vi "Voltech PM1000+ Inrush Measurement.vi"() -> ()   [LabVIEW 2015]
doc: "The purpose of this vi is to show the basic measurements that PM1000+ can make. The results are returned using the FRD command. This returns the results that are shown on the screen, in the order in which they appear on the screen. As results are selected using comms, the results are added to the bottom of the list, with the exception of harmonics, which always appear at the end of the list."
uses:
  <vilib>/Utility/error.llb/DialogType.ctl
  <instrlib>/Voltech PM1000+/Voltech PM1000+.lvlib
panel:
  in  "Reset (True)":bool=TRUE
  in  "ID Query (True)":bool=TRUE
  in  "Serial Configuration":T1={"Baud Rate"=19200, "Parity"=0, "Data Bits"=8, "Stop Bits"=10, "Flow Control"=2} {"Flow Control" items=["None"=0, "RTS/CTS"=2]; "Stop Bits" items=["1.0"=10]; "Data Bits" items=["8"=8]; "Parity" items=["None"]; "Baud Rate" items=["9600"=9600, "19200"=19200, "38400"=38400]}
  in  "Measurements":T2={"Current Range (100Apk)"=3, "Measurements - Inrush"=[2, 3, 4, 5]} {"Current Range (100Apk)" items=["0.1Apk", "0.4Apk", "1.6Apk", "6.25Apk", "25Apk", "100Apk"]}
  out "Number of Measurements":u32
  in  "Select Mode (Normal)":u16(ring)=2 items=["Normal", "Ballast", "Inrush", "Standby Power", "Integrator"]
  in  "Enable Autozero  (True)":bool=TRUE caption="Autozero  (Enable)"
  in  "Enable Blanking (True)":bool=TRUE
  in  "Shunt (Internal)":u16(ring) items=["Internal", "External"]
  in  "Freq Source (Voltage)":u16(ring) items=["Voltage", "Current"]
  in  "Fixed/Auto Ranging":T3 {"Volts Ranging (Auto)" items=["Auto", "10Vpk", "46Vpk", "215Vpk", "900Vpk"]; "Amps Ranging (Auto)" items=["Auto", "0.1Apk", "0.4Apk", "1.6Apk", "6.25Apk", "25Apk", "100Apk"]}
  in  "Scaling":T4={"Voltage Sacling (1.0000)"=1.0, "Current Sacling (1.0000)"=1.0} {"Current Sacling (1.0000)" min=1e-06 max=1000000.0 step=1.0 format="%.6f"; "Voltage Sacling (1.0000)" min=1e-06 max=1000000.0 step=1.0 format="%.6f"}
  in  "VISA resource name":refnum<visa-resource-name>
  in  "stop":bool
  out "Parameter":string[](array[string])
  out "Value":dbl[](array[numeric])
  # "(c) 2008-2009 Voltech Instruments.  ALL RIGHTS RESERVED."
  # "Configuration Side"
  # "1. Leave it as default or set up the PM1000+ instruments on the left  \n    \"Configuration Side\".\n2. Press Ctrl+R to run the test.\n3. Press the lower right side \"STOP\" button to stop the test."
  # "Results Side"
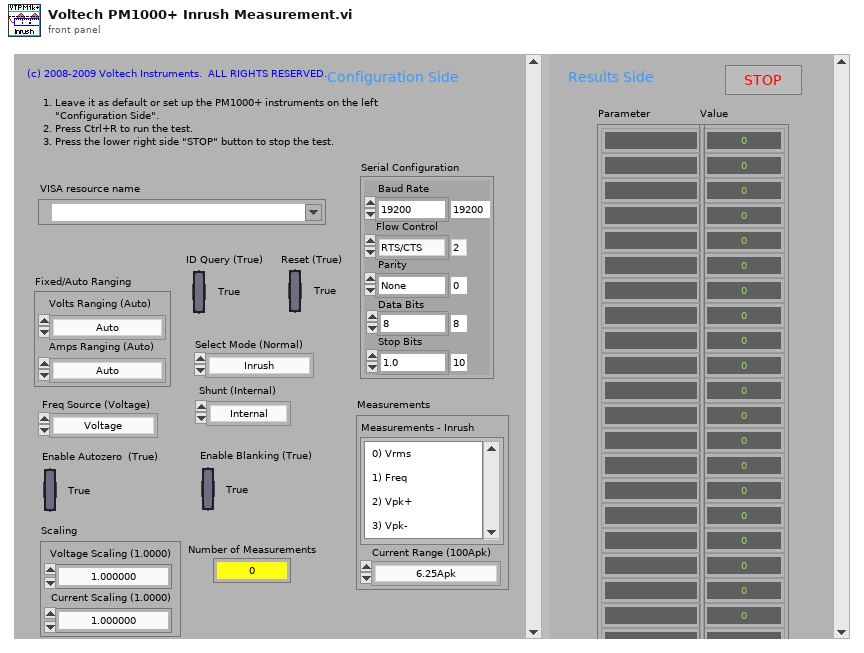
[diagram p1: front panel]
types:
  T1 = cluster{"Baud Rate":u32, "Parity":u16, "Data Bits":u16, "Stop Bits":u16, "Flow Control":u16}
  T2 = cluster{"Current Range (100Apk)":i32, "Measurements - Inrush":i32[]}
  T3 = cluster{"Amps Ranging (Auto)":u16, "Volts Ranging (Auto)":u16}
  T4 = cluster{"Voltage Sacling (1.0000)":dbl, "Current Sacling (1.0000)":dbl}
  T5 = typedef "DialogType.ctl" = u16
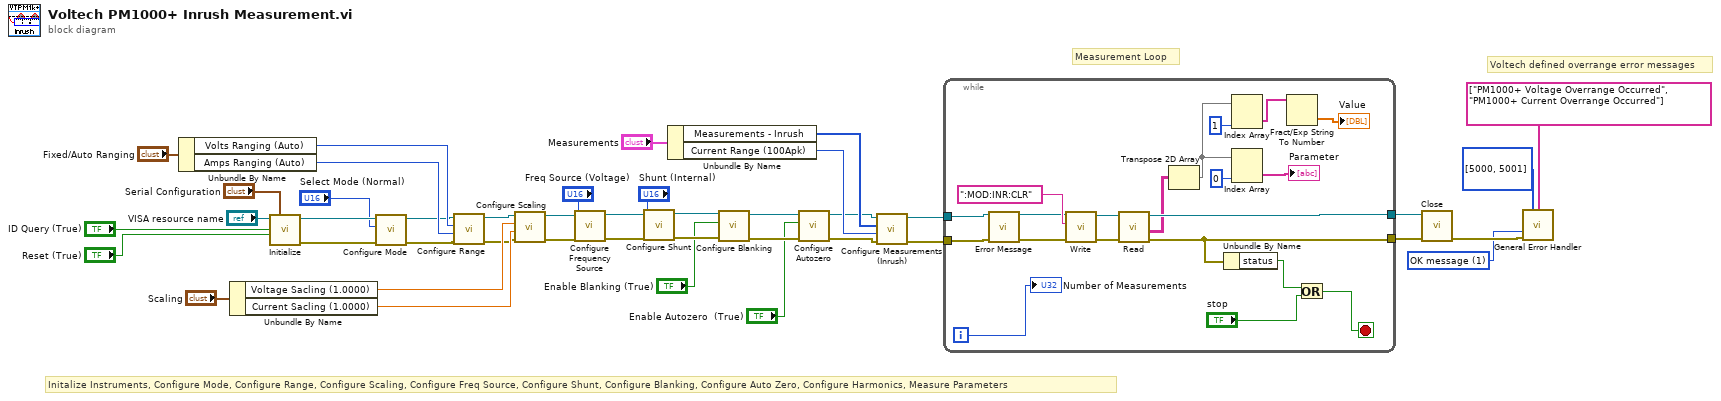
[diagram p0: block diagram]
diagram:
  w14 = T5 1 items=["no dialog", "OK message", "continue or stop message", "OK message + warnings", "continue/stop + warnings"] ("type of dialog (OK msg:1)")
  # "Voltech defined overrange error messages"
  # "Measurement Loop"
  # "Initalize Instruments, Configure Mode, Configure Range, Configure Scaling, Configure Freq Source, Configure Shunt, Configure Blanking, Configure Auto Zero, Configure Harmonics, Measure Parameters"
  n1 = Unbundle By Name("Fixed/Auto Ranging") -> ("Volts Ranging (Auto)"=w29:u16, "Amps Ranging (Auto)"=w28:u16)
  n2 = Unbundle By Name("Scaling") -> ("Voltage Sacling (1.0000)"=w32:dbl, "Current Sacling (1.0000)"=w31:dbl)
  n3 = call <instrlib>:"Initialize.vi"("Serial Configuration"="Serial Configuration", "Reset (True)"="Reset (True)", "ID Query (True)"="ID Query (True)", "VISA resource name"="VISA resource name") -> ("error out"=w6:errorcluster, "VISA resource name out"=w9:refnum<visa-resource-name>)  [unwired: 6 in]
  n4 = call <instrlib>:"Configure Mode.vi"("error in (no error)"=w6, "Select Mode (Normal)"="Select Mode (Normal)", "VISA resource name"=w9) -> ("error out"=w7:errorcluster, "VISA resource name out"=w8:refnum<visa-resource-name>)  [unwired: 7 in]
  n5 = call <instrlib>:"Configure Range.vi"("error in (no error)"=w7, "Current Range (Auto)"=w28, "Voltage Range (Auto)"=w29, "VISA resource name"=w8) -> ("error out"=w10:errorcluster, "VISA resource name out"=w11:refnum<visa-resource-name>)  [unwired: 6 in]
  n6 = call <instrlib>:"Configure Scaling.vi"("error in (no error)"=w10, "Current Sacling (1.0000)"=w31, "Voltage Sacling (1.0000)"=w32, "VISA resource name"=w11) -> ("error out"=w38:errorcluster, "VISA resource name out"=w39:refnum<visa-resource-name>)  [unwired: 6 in]
  n7 = call <instrlib>:"Configure Frequency Source.vi"("error in (no error)"=w38, "Frequency Source (Voltage)"="Freq Source (Voltage)", "VISA resource name"=w39) -> ("error out"=w41:errorcluster, "VISA resource name out"=w40:refnum<visa-resource-name>)  [unwired: 7 in]
  n8 = call <instrlib>:"Configure Shunt.vi"("error in (no error)"=w41, "Shunt (Internal)"="Shunt (Internal)", "VISA resource name"=w40) -> ("error out"=w36:errorcluster, "VISA resource name out"=w37:refnum<visa-resource-name>)  [unwired: 7 in]
  n9 = Unbundle By Name("Measurements") -> ("Measurements - Inrush"=w17:i32[], "Current Range (100Apk)"=w18:i32)
  n10 = call <instrlib>:"Configure Blanking.vi"("error in (no error)"=w36, "Enable Blanking (True)"="Enable Blanking (True)", "VISA resource name"=w37) -> ("error out"=w34:errorcluster, "VISA resource name out"=w35:refnum<visa-resource-name>)  [unwired: 7 in]
  n11 = call <instrlib>:"Configure Autozero.vi"("error in (no error)"=w34, "Enable Autozero (True)"="Enable Autozero  (True)", "VISA resource name"=w35) -> ("error out"=w12:errorcluster, "VISA resource name out"=w13:refnum<visa-resource-name>)  [unwired: 7 in]
  n12 = call <instrlib>:"Configure Measurements (Inrush).vi"("error in (no error)"=w12, "Current Range (100Apk)"=w18, "Inrush Measurements"=w17, "VISA resource name"=w13) -> ("error out"=w20:errorcluster, "VISA resource name out"=w21:refnum<visa-resource-name>)  [unwired: 6 in]
  n13 = while {
    tunnel: [w62] -> w23
    tunnel: [w46] -> w22
    tunnel: w21 -> [w48]
    tunnel: w20 -> [w47]
    i -> [w61]
    stop <- w43 stop-if-true
    n14 = call <instrlib>:"Error Message.vi"("VISA resource name"=w48, "error in (no error)"=w47) -> ("VISA resource name out"=w50:refnum<visa-resource-name>, "error out"=w49:errorcluster)  [unwired: 12 in]
    n15 = call <instrlib>:"Write.vi"("error in (no error)"=w49, "Write Buffer"=":MOD:INR:CLR", "VISA resource name"=w50) -> ("error out"=w59:errorcluster, "VISA resource name out"=w60:refnum<visa-resource-name>)  [unwired: 7 in]
    n16 = call <instrlib>:"Read.vi"("error in (no error)"=w59, "VISA resource name"=w60) -> ("error out"=w46:errorcluster, "Measurement Results"=w57:string[][], "VISA resource name out"=w62:refnum<visa-resource-name>)  [unwired: 7 in]
    n17 = Transpose 2D Array(2D array=w57) -> (transposed array=w56:string[][])
    n18 = Unbundle By Name(w46) -> ("status"=w45:bool)
    n19 = Index Array(array=w56, index (col)=1) -> (element=w53:string[])  [unwired: 1 in]
    n20 = Index Array(array=w56, index (col)=0) -> (element=→"Parameter":string[])  [unwired: 1 in]
    n21 = Fract/Exp String To Number(string=w53) -> (number=→"Value":dbl[])  [unwired: 3 in, 1 out]
    n22 = Or(x=w45, y="stop") -> (x .or. y?=w43:bool)
    "Number of Measurements" <- w61
  }
  n23 = call <instrlib>:"Close.vi"("error in (no error)"=w22, "VISA resource name"=w23) -> ("error out"=w15:errorcluster)  [unwired: 9 in]
  n24 = call <vilib>:"General Error Handler.vi"("[user-defined codes]"=i32[] [5000, 5001], "[user-defined descriptions]"=string[] ["PM1000+ Voltage Overrange Occurred", "PM1000+ Current Overrange Occurred"], "type of dialog (OK msg:1)"=w14, "error in (no error)"=w15) -> ()  [unwired: 7 in, 5 out]
